vi "HFRR ADV v02.vi"() -> ()   [LabVIEW 2023] (continued)
            n997 = local read "Sample ID"() -> (w2636:string)
            n998 = local read "Temperature after test 2"() -> (w2623:dbl)
            n999 = local read "Test Date"() -> (w2635:string)
            n1000 = local read "String 45"() -> (w2549:string)
            n1001 = local read "String 32"() -> (w2633:string)
            n1002 = local read "String 31"() -> (w2634:string)
            n1003 = local read "String 38"() -> (w2571:string)
            n1004 = local read "Humidity after test 2"() -> (w2619:dbl)
            n1005 = local read "s.NO"() -> (w2551:string)
            n1006 = local read "String 36"() -> (w2574:string)
            n1007 = local read "Temperature before test 2"() -> (w2618:dbl)
            n1008 = local read "String 37"() -> (w2577:string)
            n1009 = local read "AVP 2"() -> (w2616:dbl)
            n1010 = local read "HCF 2"() -> (w2627:dbl)
            n1011 = local read "MWSD 2"() -> (w2615:dbl)
            n1012 = local read "String 35"() -> (w2581:string)
            n1013 = local write "Export"(FALSE ("Export")) -> ()
            n1014 = local read "Humidity before test 2"() -> (w2604:dbl)
            n1015 = Concatenate Strings("7," ("string"), w2571) -> (w2572:string)
            n1016 = Concatenate Strings("6," ("string"), w2574) -> (w2575:string)
            n1017 = local read "S 39"() -> (w2582:string)
            n1018 = Concatenate Strings("5," ("string"), w2577) -> (w2578:string)
            n1019 = local read "String 34"() -> (w2586:string)
            n1020 = Concatenate Strings("4," ("string"), w2581) -> (w2580:string)
            n1021 = Concatenate Strings("3," ("string"), w2582) -> (w2584:string)
            n1022 = local read "S 38"() -> (w2589:string)
            n1023 = Number To Fractional String(number=w2627, width (-)=i16 6, precision (6)=i16 2) -> (F-format string=w2628:string)  [unwired: 1 in]
            n1024 = Number To Fractional String(number=w2615, width (-)=i16 6, precision (6)=i16 2) -> (F-format string=w2613:string)  [unwired: 1 in]
            n1025 = Number To Fractional String(number=w2616, width (-)=i16 6, precision (6)=i16 2) -> (F-format string=w2614:string)  [unwired: 1 in]
            n1026 = Number To Fractional String(number=w2623, width (-)=i16 6, precision (6)=i16 2) -> (F-format string=w2622:string)  [unwired: 1 in]
            n1027 = Number To Fractional String(number=w2619, width (-)=i16 6, precision (6)=i16 2) -> (F-format string=w2617:string)  [unwired: 1 in]
            n1028 = Number To Fractional String(number=w2618, width (-)=i16 6, precision (6)=i16 2) -> (F-format string=w2624:string)  [unwired: 1 in]
            n1029 = Number To Fractional String(number=w2604, width (-)=i16 6, precision (6)=i16 2) -> (F-format string=w2603:string)  [unwired: 1 in]
            n1030 = local read "String 39"() -> (w2568:string)
            n1031 = Concatenate Strings("2," ("string"), w2586) -> (w2585:string)
            n1032 = local read "WS1.4 2"() -> (w2631:dbl)
            n1033 = Concatenate Strings(w2561, "," ("string"), w2549, w2551, w2550, w2633, w2636, w2550, w2634, w2635, w2561) -> (w2559:string)
            n1034 = Concatenate Strings("1," ("string"), w2589) -> (w2588:string)
            n1035 = Concatenate Strings("8," ("string"), w2568) -> (w2569:string)
            n1036 = Number To Fractional String(number=w2631, precision (6)=i16 2) -> (F-format string=w2632:string)  [unwired: 2 in]
            n1037 = Concatenate Strings(w2629, w2588, w2603, w2629, w2585, w2624, w2629, w2584, w2617, w2629, w2580, w2622, w2629, w2578, w2613, w2629, w2575, w2614, w2629, w2572, w2628, w2629, w2569, w2632) -> (w2591:string)
            n1038 = Concatenate Strings("S.No," ("string"), "                                       Parameters" ("string")) -> (w2562:string)
            n1039 = local read "TITTLE"() -> (w2557:string)
            n1040 = local read "String 33"() -> (w2566:string)
            n1041 = local read "Tested by"() -> (w2565:string)
            n1042 = Concatenate Strings("=" ("string"), w2557) -> (w2556:string)
            n1043 = local read "String 29"() -> (w2598:string)
            n1044 = Concatenate Strings("," ("string"), "                                                                             " ("string")) -> (w2554:string)
            n1045 = Concatenate Strings(w2556, w2552, w2559, w2552, w2562, w2591, w2552, w2554, w2566, w2565) -> (→"export":string)
            n1046 = Match Pattern(string=w2598, regular expression=".dwm") -> (before substring=w2594:string)  [unwired: 1 in, 3 out]
            "before substring" <- w2594
            n1047 = case shown="\"xlx\"" "Select File Type" {
              tunnel: w2594 -> [w2639 w2641 w2643]
              tunnel: [w2637 w2642 w2644] -> w2593
              frame "xlx" {
                n1048 = Concatenate Strings(w2639, ".xls" ("string")) -> (w2637:string)
              }
              frame "csv" {
                n1049 = Concatenate Strings(w2641, ".csv" ("string")) -> (w2642:string)
              }
              frame "txt" {
                n1050 = Concatenate Strings(w2643, ".txt" ("string")) -> (w2644:string)
              }
            }
            n1051 = String To Path(string=w2593) -> (path=w2600:path)
            n1052 = local read "export"() -> (w2595:string)
            n1053 = call <vilib>:"Write Characters To File.vi"("append to file? (new file:F)"=FALSE, "character string"=w2595, "file path (dialog if empty)"=w2600) -> ()  [unwired: 2 in, 1 out]
          }
        }
        n1054 = case shown="True" "OK Button 16" {
          frame False {
          }
          frame True {
            n1055 = stacked-sequence {
              frame #0 {
                n1056 = local read "Numeric 16"() -> (w2759:i32)
                n1057 = local write "Numeric 10"(w2759) -> ()
              }
              frame #1 {
                n1058 = local read "String 29"() -> (w2763:string)
                n1059 = String To Path(string=w2763) -> (path=w2762:path)
                n1060 = local read "S.NO"() -> (→"s.NO":string)
                n1061 = Open/Create/Replace File "Open File"(file path (use dialog)=w2762) -> (refnum out=w2764:refnum<file>)  [unwired: 5 in, 2 out]
                n1062 = for {
                  N: 16 -> [_]
                  tunnel: w2764 -> [w2771]
                  i -> [w2767]
                  (unwired) TRUE ("line mode (F)")
                  n1063 = Read from Text File "Read File"(file (use dialog)=w2771) -> (text=w2765:string)  [unwired: 3 in, 3 out]
                  n1064 = Match Pattern(string=w2765, regular expression="(") -> (after substring=w2770:string)  [unwired: 1 in, 3 out]
                  n1065 = Match Pattern(string=w2770, regular expression=")") -> (before substring=w2766:string)  [unwired: 1 in, 3 out]
                  n1066 = case shown="1" w2767 {
                    tunnel: w2766 -> [w2772 w2773 _ _ w2774 w2775 w2776 w2778 w2780 w2782 w2784 w2786 w2788 w2790 _]
                    tunnel: w2765 -> [_ _ _ _ _ _ _ _ _ _ _ _ _ _ _]
                    frame 0 {
                      "TITTLE" <- w2772
                    }
                    frame 1 {
                      "Sample ID" <- w2773
                    }
                    frame 2 {
                    }
                    frame 3 {
                    }
                    frame 4 {
                      "Test Date" <- w2774
                    }
                    frame 5 {
                      "Tested by" <- w2775
                    }
                    frame 6 {
                      n1067 = Fract/Exp String To Number(string=w2776) -> (number=→"Humidity before test 2":dbl)  [unwired: 3 in, 1 out]
                    }
                    frame 7 {
                      n1068 = Fract/Exp String To Number(string=w2778) -> (number=→"Temperature before test 2":dbl)  [unwired: 3 in, 1 out]
                    }
                    frame 8 {
                      n1069 = Fract/Exp String To Number(string=w2780) -> (number=→"Humidity after test 2":dbl)  [unwired: 3 in, 1 out]
                    }
                    frame 9 {
                      n1070 = Fract/Exp String To Number(string=w2782) -> (number=→"Temperature after test 2":dbl)  [unwired: 3 in, 1 out]
                    }
                    frame 10 {
                      n1071 = Fract/Exp String To Number(string=w2784) -> (number=→"MWSD 2":dbl)  [unwired: 3 in, 1 out]
                    }
                    frame 11 {
                      n1072 = Fract/Exp String To Number(string=w2786) -> (number=→"AVP 2":dbl)  [unwired: 3 in, 1 out]
                    }
                    frame 12 {
                      n1073 = Fract/Exp String To Number(string=w2788) -> (number=→"HCF 2":dbl)  [unwired: 3 in, 1 out]
                    }
                    frame 13 {
                      n1074 = Fract/Exp String To Number(string=w2790) -> (number=→"WS1.4 2":dbl)  [unwired: 3 in, 1 out]
                    }
                    frame 14, Default {
                    }
                  }
                }
              }
              frame #2 {
              }
            }
            n1075 = local write "OK Button 16"(FALSE ("OK Button 13")) -> ()
          }
        }
        n1076 = call <vilib>:"Query Available Printers.vi"() -> ("system configured printers"=w2434:string[])  [unwired: 9 in, 2 out]
        "System Configured Printers 2" <- w2434
        n1077 = Index Array(array=w2434, index="Select Printer 3") -> (element=w2436:string)
        "Selected Printer" <- w2436
        n1078 = local read "OK Button 16"() -> (w2430:bool)
        n1079 = case shown="True" "Print" {
          tunnel: w2436 -> [_ w2728]
          frame False {
          }
          frame True {
            (unwired) i16 6 ("width (-)")
            (unwired) "TESTED BY : "
            (unwired) "TESTED DATE :"
            (unwired) "SAMPLE ID : "
            (unwired) "SAMPLE DESIGN : "
            w2686 = "\r"
            w2703 = "\r"
            # "add image"
            n1080 = local read "String 45"() -> (w2646:string)
            n1081 = local read "Sample ID"() -> (w2676:string)
            n1082 = local read "Tested by"() -> (w2679:string)
            n1083 = local read "Test Date"() -> (w2677:string)
            n1084 = local read "String 32"() -> (w2681:string)
            n1085 = local read "String 31"() -> (w2680:string)
            n1086 = local read "String 33"() -> (w2682:string)
            n1087 = local read "s.NO"() -> (w2647:string)
            n1088 = call <vilib>:"New Report.vi"("report type"=enum16{"Standard Report", "HTML"}."Standard Report") -> ("report out"=w2726:refnum<class "NI_report.lvclass">, "error out"=w2725:errorcluster)  [unwired: 13 in]
            n1089 = local read "TITTLE"() -> (w2678:string)
            n1090 = call-dynamic "Set Report Header Text.vi"("report in"=w2726, "center header text"=w2678, "error in (no error)"=w2725) -> ("report out"=w2697:refnum<class "NI_report.lvclass">, "error out"=w2698:errorcluster)  [unwired: 11 in]
            n1091 = Concatenate Strings(w2703, w2646, w2647, w2703, w2681, w2676, w2703, w2680, w2677, w2703, w2682, w2679, w2703) -> (w2696:string)
            "test by" <- w2696
            n1092 = local read "Temperature after test 2"() -> (w2692:dbl)
            n1093 = local read "String 38"() -> (w2652:string)
            n1094 = local read "Humidity after test 2"() -> (w2701:dbl)
            n1095 = local read "String 36"() -> (w2656:string)
            n1096 = local read "Temperature before test 2"() -> (w2702:dbl)
            n1097 = local read "String 37"() -> (w2659:string)
            n1098 = local read "AVP 2"() -> (w2705:dbl)
            n1099 = local read "HCF 2"() -> (w2688:dbl)
            n1100 = local read "MWSD 2"() -> (w2706:dbl)
            n1101 = local read "String 35"() -> (w2661:string)
            n1102 = call-poly <vilib>:"Append Report Text.vi"("report in"=w2697, "text"=w2696, "error in (no error)"=w2698) -> ("report out"=w2700:refnum<class "NI_report.lvclass">, "error out"=w2699:errorcluster)  [unwired: 9 in, 2 out]
            n1103 = local read "Humidity before test 2"() -> (w2717:dbl)
            n1104 = Concatenate Strings("7)" ("string"), w2652) -> (w2653:string)
            n1105 = local read "S 39"() -> (w2664:string)
            n1106 = local read "String 34"() -> (w2666:string)
            n1107 = Concatenate Strings("6)" ("string"), w2656) -> (w2655:string)
            n1108 = Concatenate Strings("5)" ("string"), w2659) -> (w2658:string)
            n1109 = Concatenate Strings("4)" ("string"), w2661) -> (w2662:string)
            n1110 = Concatenate Strings("3)" ("string"), w2664) -> (w2665:string)
            n1111 = local read "S 38"() -> (w2671:string)
            n1112 = Concatenate Strings("2)" ("string"), w2666) -> (w2667:string)
            n1113 = Number To Fractional String(number=w2688, width (-)=i16 6, precision (6)=i16 2) -> (F-format string=w2687:string)  [unwired: 1 in]
            n1114 = Number To Fractional String(number=w2706, width (-)=i16 6, precision (6)=i16 2) -> (F-format string=w2708:string)  [unwired: 1 in]
            n1115 = Number To Fractional String(number=w2705, width (-)=i16 6, precision (6)=i16 2) -> (F-format string=w2707:string)  [unwired: 1 in]
            n1116 = Number To Fractional String(number=w2692, width (-)=i16 6, precision (6)=i16 2) -> (F-format string=w2693:string)  [unwired: 1 in]
            n1117 = Number To Fractional String(number=w2701, width (-)=i16 6, precision (6)=i16 2) -> (F-format string=w2704:string)  [unwired: 1 in]
            n1118 = Number To Fractional String(number=w2702, width (-)=i16 6, precision (6)=i16 2) -> (F-format string=w2691:string)  [unwired: 1 in]
            n1119 = Number To Fractional String(number=w2717, width (-)=i16 6, precision (6)=i16 2) -> (F-format string=w2722:string)  [unwired: 1 in]
            n1120 = call-poly <vilib>:"Append Report Text.vi"("report in"=w2700, "error in (no error)"=w2699) -> ("report out"=w2721:refnum<class "NI_report.lvclass">, "error out"=w2719:errorcluster)  [unwired: 10 in, 2 out]
            n1121 = local read "String 39"() -> (w2649:string)
            n1122 = local read "WS1.4 2"() -> (w2684:dbl)
            n1123 = Concatenate Strings("1)" ("string"), w2671) -> (w2670:string)
            n1124 = Concatenate Strings("8)" ("string"), w2649) -> (w2650:string)
            n1125 = Number To Fractional String(number=w2684, precision (6)=i16 2) -> (F-format string=w2683:string)  [unwired: 2 in]
            n1126 = Concatenate Strings(w2686, w2670, w2722, w2686, w2667, w2691, w2686, w2665, w2704, w2686, w2662, w2693, w2686, w2658, w2708, w2686, w2655, w2707, w2686, w2653, w2687, w2686, w2650, w2683) -> (w2674:string)
            "export 2" <- w2674
            n1127 = call-poly <vilib>:"Append Report Text.vi"("report in"=w2721, "text"=w2674, "error in (no error)"=w2719) -> ("report out"=w2720:refnum<class "NI_report.lvclass">, "error out"=w2718:errorcluster)  [unwired: 9 in, 2 out]
            n1128 = call-dynamic "Print Report.vi"("report in"=w2720, "printer name (default)"=w2728, "error in (no error)"=w2718) -> ("report out"=w2730:refnum<class "NI_report.lvclass">, "error out"=w2731:errorcluster)  [unwired: 11 in]
            n1129 = local read "test by"() -> (w2673:string)
            n1130 = local read "TITTLE"() -> (w2675:string)
            n1131 = local write "Print"(FALSE ("Print FF")) -> ()
            n1132 = call-dynamic "Dispose Report.vi"("report in"=w2730, "error in (no error)"=w2731) -> ()  [unwired: 13 in, 1 out]
            n1133 = Concatenate Strings(w2675, w2674, w2673) -> (→"output":string)
          }
        }
        n1134 = case shown="True" w2430 {
          frame False {
          }
          frame True {
            n1135 = flat-sequence {
              frame #0 {
              }
              frame #1 {
                n1136 = Wait (ms)(milliseconds to wait=u32 100) -> ()  [unwired: 1 out]
              }
              frame #2 {
                n1137 = local write "OK Button 16"(FALSE ("Print 3")) -> ()
              }
            }
          }
        }
        n1138 = case shown="True" "OK Button 17" {
          frame False {
          }
          frame True {
            (unwired) 0  # existing file
            w2745 = "Choose a datalog file to open"  # prompt
            n1139 = local read "String"() -> (w2740:string)
            n1140 = local write "OK Button 17"(FALSE ("OK Button 17")) -> ()
            n1141 = String To Path(string=w2740) -> (path=w2741:path)
            n1142 = File Dialog(6:"*.duf" ("pattern"), 7:w2745, 11:w2741) -> (0:w2732:errorcluster, 3:w2751:path)  [unwired: 4 in, 2 out]
            n1143 = Unbundle(w2732) -> ()  [unwired: 3 out]
            n1144 = Open/Create/Replace File "Open File"(file path (use dialog)=w2751) -> (refnum out=w2743:refnum<file>)  [unwired: 5 in, 2 out]
            n1145 = Path To String(path=w2751) -> (string=w2734:string)
            n1146 = while {
              tunnel: w2743 -> [w2755]
              i -> [w2752]
              stop <- w2753 continue-if-true
              (unwired) TRUE ("line mode (F)")
              n1147 = local write "Numeric 16"(w2752) -> ()
              n1148 = Read from Text File "Read File"(file (use dialog)=w2755) -> (text=w2754:string)  [unwired: 3 in, 3 out]
              n1149 = String Length(string=w2754) -> (length=w2757:i32)
              n1150 = Greater?(x=w2757, y=1) -> (0:w2753:bool)
            }
            n1151 = local write "String 29"(w2734) -> ()
            n1152 = Match Pattern(string=w2734, regular expression=".dwm" ("substring (\"\")")) -> (before substring=w2735:string)  [unwired: 1 in, 3 out]
            "String Indicator 3" <- w2735
            n1153 = Search and Replace String(input string=w2734, search string=".duf", replace string=".dgf" ("replace string (\"\")")) -> (result string=→"String Indicator 4":string)  [unwired: 5 in, 3 out]
            n1154 = String To Path(string=w2735) -> (path=w2742:path)
            "path" <- w2742
            n1155 = Strip Path(path=w2751) -> (name=w2749:string)  [unwired: 1 out]
            n1156 = call <vilib>:"Read Characters From File.vi"("file path (dialog if empty)"=w2742, "start of read offset (chars.:0)"=60 ("start of read offset (chars.: 0)")) -> ("character string"=→"String Indicator 2":string)  [unwired: 4 in, 3 out]
            n1157 = Match Pattern(string=w2749, regular expression=".dwm") -> (before substring=w2733:string)  [unwired: 1 in, 3 out]
            "String Indicator" <- w2733
            n1158 = local write "TITTLE 2"(w2733) -> ()
          }
        }
        n1159 = case shown="True" "Print 2" {
          frame False {
          }
          frame True {
            n1160 = flat-sequence {
              frame #0 {
                n1161 = local read "Ref A Test Date :"() -> (→"TITTLE 4":string)
                n1162 = local read "Sample ID"() -> (→"Sample ID  2":string)
                n1163 = local read "s.NO"() -> (→"s.NO 2":string)
                n1164 = local read "Test Date"() -> (→"Test Date 2":string)
                n1165 = local read "Tested by"() -> (→"Tested by 2":string)
                n1166 = local read "Temperature before test 3"() -> (w2454:dbl)
                n1167 = local read "Temperature before test 3"() -> (→"Temperature after test 5":dbl)
                n1168 = local read "Temperature after test 3"() -> (→"Temperature after test 4":dbl)
                n1169 = local read "Sample ID  3"() -> (→"Sample ID  6":string)
                n1170 = local read "Sample ID  4"() -> (→"Sample ID  7":string)
                n1171 = local read "Humidity before test 3"() -> (→"Humidity before test 4":dbl)
                n1172 = local read "Humidity after test 3"() -> (→"Humidity after test 4":dbl)
                n1173 = local write "Temperature before test 3"(w2454) -> ()
                n1174 = String To Path(string="C:\\LAB-IQ-NXT\\im\\Temp_resized.jpg") -> (path=w2446:path)
                "path 2" <- w2446
                n1175 = local read "image data"() -> (w2445:T8)
                n1176 = Wait (ms)(milliseconds to wait=u32 20) -> ()  [unwired: 1 out]
                n1177 = call <vilib>:"Write JPEG File.vi"("image data"=w2445, "path to JPEG file"=w2446) -> ()  [unwired: 8 in, 2 out]
                "Ref A Test Date :" <- "Ref A Test Date :"
                "Ref B Test Date :" <- "Ref B Test Date :"
                "Ref B Scar Value :" <- "Ref B Scar Value :"
                "Ref A Scar Value :" <- "Ref A Scar Value :"
              }
              frame #1 {
                (unwired) HTML_Report_Image_Alignment."MIDDLE" ("alignment (default)")
                w2482 = u16 0 items=["portrait", "landscape"] ("orientation (portrait)")
                (unwired) HTML_Report_Image_Alignment."ABSMIDDLE" ("alignment (default)")
                (unwired) "TESTED BY : "
                (unwired) "TESTED DATE :"
                (unwired) "SAMPLE ID : "
                (unwired) "SAMPLE DESIGN : "
                w2515 = "\r"
                # "add image"
                n1178 = call <vilib>:"New Report.vi"("report type"=enum16{"Standard Report", "HTML"}."HTML") -> ("report out"=w2486:refnum<class "NI_report.lvclass">, "error out"=w2484:errorcluster)  [unwired: 13 in]
                n1179 = Wait (ms)(milliseconds to wait=u32 20) -> ()  [unwired: 1 out]
                n1180 = call-dynamic "Set Report Orientation.vi"("report in"=w2486, "orientation (portrait)"=w2482, "error in (no error)"=w2484) -> ("report out"=w2485:refnum<class "NI_report.lvclass">, "error out"=w2483:errorcluster)  [unwired: 11 in]
                n1181 = for {
                  N: 5 -> [_]
                  tunnel: w2485 -> [w2536]
                  tunnel: [w2535] -> w2464
                  tunnel: w2483 -> [w2534]
                  tunnel: [w2533] -> w2463
                  n1182 = call-dynamic "Set Report Tab Width.vi"("report in"=w2536, "error in (no error)"=w2534) -> ("report out"=w2535:refnum<class "NI_report.lvclass">, "error out"=w2533:errorcluster)  [unwired: 12 in]
                }
                n1183 = local read "Sample ID  2"() -> (w2508:string)
                n1184 = local read "s.NO 2"() -> (w2507:string)
                n1185 = local read "Test Date 2"() -> (w2509:string)
                n1186 = local read "Tested by 2"() -> (w2510:string)
                n1187 = local read "String 46"() -> (w2506:string)
                n1188 = local read "String 48"() -> (w2512:string)
                n1189 = local read "String 47"() -> (w2511:string)
                n1190 = local read "String 49"() -> (w2513:string)
                n1191 = local read "TITTLE"() -> (w2481:string)
                n1192 = call-dynamic "Set Report Header Text.vi"("report in"=w2464, "center header text"=w2481, "error in (no error)"=w2463) -> ("report out"=w2502:refnum<class "NI_report.lvclass">, "error out"=w2501:errorcluster)  [unwired: 11 in]
                n1193 = for {
                  N: 1 -> [_]
                  tunnel: [w2540] -> w2488
                  tunnel: [w2539] -> w2487
                  tunnel: w2502 -> [w2538]
                  tunnel: w2501 -> [w2537]
                  n1194 = call-dynamic "New Report Line.vi"("report in"=w2538, "error in (no error)"=w2537) -> ("report out"=w2540:refnum<class "NI_report.lvclass">, "error out"=w2539:errorcluster)  [unwired: 12 in]
                }
                n1195 = for {
                  N: 2 -> [_]
                  tunnel: [w2532] -> w2494
                  tunnel: [w2531] -> w2493
                  tunnel: w2488 -> [w2530]
                  tunnel: w2487 -> [w2529]
                  n1196 = call-dynamic "New Report Line.vi"("report in"=w2530, "error in (no error)"=w2529) -> ("report out"=w2532:refnum<class "NI_report.lvclass">, "error out"=w2531:errorcluster)  [unwired: 12 in]
                }
                n1197 = Concatenate Strings(w2515, w2506, w2507, w2515, w2512, w2508, w2515, w2511, w2509, w2515, w2513, w2510, w2515) -> (→"test by 2":string)
                n1198 = for {
                  N: 25 -> [_]
                  tunnel: w2494 -> [w2528]
                  tunnel: w2493 -> [w2526]
                  tunnel: [w2527] -> w2497
                  tunnel: [w2525] -> w2496
                  n1199 = call-dynamic "Set Report Tab Width.vi"("report in"=w2528, "error in (no error)"=w2526) -> ("report out"=w2527:refnum<class "NI_report.lvclass">, "error out"=w2525:errorcluster)  [unwired: 12 in]
                }
                n1200 = control-ref of="Tab Control 9"() -> (w2492:refnum<vi>)
                n1201 = local read "Wear Scar X"() -> (w2480:dbl)
                "Length ( microns ) 2" <- w2480
                n1202 = local read "Wear Scar Y"() -> (w2479:dbl)
                "Wear Scar Y ( microns ) :" <- w2479
                n1203 = call-dynamic "Append Control Image to Report.vi"("report in"=w2497, "alignment (default)"=HTML_Report_Image_Alignment."ABSMIDDLE", "ctrl reference"=w2492, "error in (no error)"=w2496) -> ("report out"=w2491:refnum<class "NI_report.lvclass">, "error out"=w2490:errorcluster)  [unwired: 8 in, 2 out]
                n1204 = for {
                  N: 3 -> [_]
                  tunnel: [w2524] -> w2475
                  tunnel: [w2523] -> w2474
                  tunnel: w2491 -> [w2522]
                  tunnel: w2490 -> [w2521]
                  n1205 = call-dynamic "New Report Line.vi"("report in"=w2522, "error in (no error)"=w2521) -> ("report out"=w2524:refnum<class "NI_report.lvclass">, "error out"=w2523:errorcluster)  [unwired: 12 in]
                }
                n1206 = Add(x=w2480, y=w2479) -> (x+y=w2478:dbl)
                n1207 = Divide(x=w2478, y=2.0) -> (x/y=→"Mean Wear ( microns) :":dbl)
                n1208 = for {
                  N: 100 -> [_]
                  tunnel: w2475 -> [w2520]
                  tunnel: w2474 -> [w2518]
                  tunnel: [w2519] -> w2471
                  tunnel: [w2517] -> w2469
                  n1209 = call-dynamic "Set Report Tab Width.vi"("report in"=w2520, "error in (no error)"=w2518) -> ("report out"=w2519:refnum<class "NI_report.lvclass">, "error out"=w2517:errorcluster)  [unwired: 12 in]
                }
                n1210 = local read "String 10"() -> (w2466:string)
                n1211 = Concatenate Strings("C:\\LAB-IQ-NXT\\Data\\" ("string"), w2466, ".jpg" ("string")) -> ()  [unwired: 1 out]
                n1212 = String To Path(string="C:\\LAB-IQ-NXT\\im\\Temp_resized.jpg") -> (path=w2461:path)
                n1213 = call-poly <vilib>:"Append Image to Report.vi"("report in"=w2471, "path or URL of image"=w2461, "error in (no error)"=w2469) -> ("report out"=w2470:refnum<class "NI_report.lvclass">, "error out"=w2468:errorcluster)  [unwired: 9 in, 2 out]
                n1214 = call-poly <vilib>:"Open HTML Report in Browser.vi"("report in"=w2470, "error in (no error)"=w2468) -> ("report out"=w2505:refnum<class "NI_report.lvclass">, "error out"=w2504:errorcluster)  [unwired: 11 in, 1 out]
                n1215 = call-dynamic "Dispose Report.vi"("report in"=w2505, "error in (no error)"=w2504) -> ()  [unwired: 13 in, 1 out]
              }
              frame #2 {
              }
              frame #3 {
                n1216 = case shown="True" "Case Constant\n(See Context Help) 16" {
                  frame False {
                  }
                  frame True {
                    n1217 = local read "String 10"() -> (w2546:string)
                    n1218 = Concatenate Strings("C:\\LAB-IQ-NXT\\Data\\" ("string"), w2546, ".jpg" ("string")) -> (w2544:string)
                    n1219 = String To Path(string=w2544) -> (path=w2543:path)
                    n1220 = Delete(path (use dialog)=w2543) -> ()  [unwired: 4 in, 3 out]
                  }
                }
                n1221 = local write "Print 2"(FALSE ("Print")) -> ()
              }
            }
          }
        }
      }
    }
    n1222 = local read "OK Button 16"() -> (w788:bool)
    n1223 = Or(x=w788, y="OPEN") -> (x .or. y?=w789:bool)
    n1224 = case shown="True" w789 {
      tunnel: w788 -> [_ w841]
      frame False {
      }
      frame True {
        n1225 = stacked-sequence {
          tunnel: w841 -> [_ w908 _ _]
          frame #0 {
            w857 = "  " ("String 6")
            n1226 = local write "OPEN"(FALSE ("open")) -> ()
            n1227 = property on="OPEN" class="Bool (strict)"("Visible"=FALSE) -> ()  [unwired: 2 in, 2 out]
            n1228 = local write "String 12"(w857) -> ()
            n1229 = local write "String 6"(w857) -> ()
            n1230 = local write "String 7"(w857) -> ()
            n1231 = local write "String 8"(w857) -> ()
            n1232 = local read "OK Button 16"() -> (w842:bool)
            n1233 = case shown="True" w842 {
              tunnel: [w858 w859] -> w846
              frame False {
                n1234 = local read "string1"() -> (w858:string)
              }
              frame True {
                n1235 = local read "String Indicator 4"() -> (w859:string)
              }
            }
            n1236 = local read "string1 2"() -> (w845:string)
            n1237 = local read "string1 4"() -> (w843:string)
            n1238 = local read "string1 3"() -> (w844:string)
            n1239 = String To Path(string=w846) -> (path=w854:path)
            n1240 = String To Path(string=w845) -> (path=w853:path)
            n1241 = String To Path(string=w844) -> (path=w852:path)
            n1242 = String To Path(string=w843) -> (path=w851:path)
            n1243 = Open/Create/Replace File "Open File"(file path (use dialog)=w854) -> (refnum out=w850:refnum<file>)  [unwired: 5 in, 2 out]
            n1244 = Open/Create/Replace File "Open File"(file path (use dialog)=w853) -> (refnum out=w849:refnum<file>)  [unwired: 5 in, 2 out]
            n1245 = Open/Create/Replace File "Open File"(file path (use dialog)=w852) -> (refnum out=w848:refnum<file>)  [unwired: 5 in, 2 out]
            n1246 = Open/Create/Replace File "Open File"(file path (use dialog)=w851) -> (refnum out=w847:refnum<file>)  [unwired: 5 in, 2 out]
            n1247 = while {
              tunnel: w850 -> [w865]
              i -> [w861]
              stop <- w860 continue-if-true
              (unwired) TRUE ("line mode (F)")
              n1248 = Read from Text File "Read File"(file (use dialog)=w865) -> (text=w862:string)  [unwired: 3 in, 3 out]
              n1249 = local write "Numeric 8"(w861) -> ()
              n1250 = String Length(string=w862) -> (length=w864:i32)
              n1251 = Greater?(x=w864, y=1) -> (0:w860:bool)
            }
            n1252 = while {
              tunnel: w849 -> [w871]
              i -> [w867]
              stop <- w866 continue-if-true
              (unwired) TRUE ("line mode (F)")
              n1253 = Read from Text File "Read File"(file (use dialog)=w871) -> (text=w868:string)  [unwired: 3 in, 3 out]
              n1254 = local write "Numeric 11"(w867) -> ()
              n1255 = String Length(string=w868) -> (length=w870:i32)
              n1256 = Greater?(x=w870, y=1) -> (0:w866:bool)
            }
            n1257 = while {
              tunnel: w848 -> [w877]
              i -> [w873]
              stop <- w872 continue-if-true
              (unwired) TRUE ("line mode (F)")
              n1258 = Read from Text File "Read File"(file (use dialog)=w877) -> (text=w874:string)  [unwired: 3 in, 3 out]
              n1259 = local write "Numeric 12"(w873) -> ()
              n1260 = String Length(string=w874) -> (length=w876:i32)
              n1261 = Greater?(x=w876, y=1) -> (0:w872:bool)
            }
            n1262 = while {
              tunnel: w847 -> [w883]
              i -> [w879]
              stop <- w878 continue-if-true
              (unwired) TRUE ("line mode (F)")
              n1263 = Read from Text File "Read File"(file (use dialog)=w883) -> (text=w880:string)  [unwired: 3 in, 3 out]
              n1264 = local write "Numeric 13"(w879) -> ()
              n1265 = String Length(string=w880) -> (length=w882:i32)
              n1266 = Greater?(x=w882, y=1) -> (0:w878:bool)
            }
          }
          frame #1 {
            w1035 = FALSE ("ACTUAL   MERGE")
            # "Sample Temp"
            # "ECR"
            # "COF"
            # "Time\nCOF\nFF\nTemp"
            n1267 = case shown="True" w908 {
              tunnel: [w1055 w1056] -> w909
              frame False {
                n1268 = local read "string1"() -> (w1055:string)
              }
              frame True {
                n1269 = local read "String Indicator 4"() -> (w1056:string)
              }
            }
            n1270 = local read "string1 2"() -> (w954:string)
            n1271 = local read "string1 4"() -> (w952:string)
            n1272 = local read "string1 3"() -> (w953:string)
            n1273 = String To Path(string=w952) -> (path=w1046:path)
            n1274 = String To Path(string=w954) -> (path=w1052:path)
            n1275 = String To Path(string=w909) -> (path=w1040:path)
            n1276 = Open/Create/Replace File "Open File"(file path (use dialog)=w1046) -> (refnum out=w1045:refnum<file>, error out=w1044:errorcluster)  [unwired: 5 in, 1 out]
            n1277 = Open/Create/Replace File "Open File"(file path (use dialog)=w1040) -> (refnum out=w1054:refnum<file>, error out=w1053:errorcluster)  [unwired: 5 in, 1 out]
            n1278 = Open/Create/Replace File "Open File"(file path (use dialog)=w1052) -> (refnum out=w1050:refnum<file>, error out=w1049:errorcluster)  [unwired: 5 in, 1 out]
            n1279 = String To Path(string=w953) -> (path=w1051:path)
            n1280 = local read "Numeric 8"() -> (w1039:i32)
            n1281 = Open/Create/Replace File "Open File"(file path (use dialog)=w1051) -> (refnum out=w1047:refnum<file>, error out=w1048:errorcluster)  [unwired: 5 in, 1 out]
            n1282 = local read "Numeric 13"() -> (w1038:i32)
            n1283 = local read "Numeric 11"() -> (w1036:i32)
            n1284 = local read "Numeric 12"() -> (w1037:i32)
            n1285 = for {
              N: w1036 -> [_]
              tunnel: w1050 -> [w1165]
              tunnel: w1049 -> [w1164]
              tunnel: [w1154] -> w1016 mode=indexing
              tunnel: [w1152] -> w1014 mode=indexing
              tunnel: [w1153] -> w1009 mode=indexing
              tunnel: w1035 -> [_]
              tunnel: [w1146] -> w1011 mode=indexing
              tunnel: [w1142] -> w987 mode=indexing
              tunnel: [w1138] -> w962 mode=indexing
              tunnel: [w1134] -> w943 mode=indexing
              tunnel: [w1129] -> w901 mode=indexing
              (unwired) TRUE ("line mode (F)")
              n1286 = Read from Text File "Read File"(file (use dialog)=w1165, error in=w1164) -> (text=w1130:string)  [unwired: 2 in, 3 out]
              n1287 = String Subset(string=w1130, offset (0)=0, length (rest)=14 ("length (rest)")) -> (substring=w1158:string)
              n1288 = Fract/Exp String To Number(string=w1158) -> (number=w1154:dbl)  [unwired: 3 in, 1 out]
              n1289 = local write "String 7"(w1130) -> ()
              n1290 = String Subset(string=w1130, offset (0)=15, length (rest)=9 ("length (rest)")) -> (substring=w1161:string)
              n1291 = Fract/Exp String To Number(string=w1161) -> (number=w1152:dbl)  [unwired: 3 in, 1 out]
              n1292 = String Subset(string=w1130, offset (0)=65, length (rest)=9 ("length (rest)")) -> (substring=w1147:string)
              n1293 = Fract/Exp String To Number(string=w1147) -> (number=w1150:dbl)  [unwired: 3 in, 1 out]
              n1294 = Add(x=w1150, y=0.0) -> (x+y=w1146:dbl)
              n1295 = String Subset(string=w1130, offset (0)=35, length (rest)=9 ("length (rest)")) -> (substring=w1155:string)
              n1296 = Fract/Exp String To Number(string=w1155) -> (number=w1153:dbl)  [unwired: 3 in, 1 out]
              n1297 = String Subset(string=w1130, offset (0)=45, length (rest)=9 ("length (rest)")) -> (substring=w1143:string)
              n1298 = Fract/Exp String To Number(string=w1143) -> (number=w1142:dbl)  [unwired: 3 in, 1 out]
              n1299 = String Subset(string=w1130, offset (0)=55, length (rest)=9 ("length (rest)")) -> (substring=w1141:string)
              n1300 = Fract/Exp String To Number(string=w1141) -> (number=w1138:dbl)  [unwired: 3 in, 1 out]
              n1301 = String Subset(string=w1130, offset (0)=25, length (rest)=9 ("length (rest)")) -> (substring=w1135:string)
              n1302 = Fract/Exp String To Number(string=w1135) -> (number=w1134:dbl)  [unwired: 3 in, 1 out]
              n1303 = String Subset(string=w1130, offset (0)=85, length (rest)=9 ("length (rest)")) -> (substring=w1133:string)
              n1304 = Fract/Exp String To Number(string=w1133) -> (number=w1129:dbl)  [unwired: 3 in, 1 out]
            }
            n1305 = for {
              N: w1037 -> [_]
              tunnel: w1048 -> [w1128]
              tunnel: w1047 -> [w1127]
              tunnel: [w1117] -> w1006 mode=indexing
              tunnel: [w1115] -> w1004 mode=indexing
              tunnel: [w1116] -> w1000 mode=indexing
              tunnel: w1035 -> [_]
              tunnel: [w1109] -> w1002 mode=indexing
              tunnel: [w1105] -> w984 mode=indexing
              tunnel: [w1101] -> w960 mode=indexing
              tunnel: [w1098] -> w941 mode=indexing
              tunnel: [w1094] -> w900 mode=indexing
              (unwired) 9 ("length (rest)")
              (unwired) 9 ("length (rest)")
              (unwired) TRUE ("line mode (F)")
              n1306 = Read from Text File "Read File"(file (use dialog)=w1127, error in=w1128) -> (text=w1095:string)  [unwired: 2 in, 3 out]
              n1307 = String Subset(string=w1095, offset (0)=0, length (rest)=14 ("length (rest)")) -> (substring=w1121:string)
              n1308 = Fract/Exp String To Number(string=w1121) -> (number=w1117:dbl)  [unwired: 3 in, 1 out]
              n1309 = local write "String 8"(w1095) -> ()
              n1310 = String Subset(string=w1095, offset (0)=15, length (rest)=9 ("length (rest)")) -> (substring=w1124:string)
              n1311 = Fract/Exp String To Number(string=w1124) -> (number=w1115:dbl)  [unwired: 3 in, 1 out]
              n1312 = String Subset(string=w1095, offset (0)=65, length (rest)=9 ("length (rest)")) -> (substring=w1114:string)
              n1313 = Fract/Exp String To Number(string=w1114) -> (number=w1111:dbl)  [unwired: 3 in, 1 out]
              n1314 = Add(x=w1111, y=0.0) -> (x+y=w1109:dbl)
              n1315 = String Subset(string=w1095, offset (0)=35, length (rest)=9 ("length (rest)")) -> (substring=w1118:string)
              n1316 = Fract/Exp String To Number(string=w1118) -> (number=w1116:dbl)  [unwired: 3 in, 1 out]
              n1317 = String Subset(string=w1095, offset (0)=45, length (rest)=9 ("length (rest)")) -> (substring=w1108:string)
              n1318 = Fract/Exp String To Number(string=w1108) -> (number=w1105:dbl)  [unwired: 3 in, 1 out]
              n1319 = String Subset(string=w1095, offset (0)=55, length (rest)=9 ("length (rest)")) -> (substring=w1103:string)
              n1320 = Fract/Exp String To Number(string=w1103) -> (number=w1101:dbl)  [unwired: 3 in, 1 out]
              n1321 = String Subset(string=w1095, offset (0)=25) -> (substring=w1099:string)  [unwired: 1 in]
              n1322 = Fract/Exp String To Number(string=w1099) -> (number=w1098:dbl)  [unwired: 3 in, 1 out]
              n1323 = String Subset(string=w1095, offset (0)=85) -> (substring=w1097:string)  [unwired: 1 in]
              n1324 = Fract/Exp String To Number(string=w1097) -> (number=w1094:dbl)  [unwired: 3 in, 1 out]
            }
            n1325 = for {
              N: w1038 -> [_]
              tunnel: w1045 -> [w1093]
              tunnel: w1044 -> [w1092]
              tunnel: [w1082] -> w998 mode=indexing
              tunnel: [w1081] -> w991 mode=indexing
              tunnel: w1035 -> [_]
              tunnel: [w1070] -> w996 mode=indexing
              tunnel: [w1075] -> w993 mode=indexing
              tunnel: [w1071] -> w983 mode=indexing
              tunnel: [w1066] -> w958 mode=indexing
              tunnel: [w1062] -> w939 mode=indexing
              tunnel: [w1057] -> w899 mode=indexing
              (unwired) 1.0 ("x")
              (unwired) TRUE ("line mode (F)")
              n1326 = Read from Text File "Read File"(file (use dialog)=w1093, error in=w1092) -> (text=w1058:string)  [unwired: 2 in, 3 out]
              n1327 = String Subset(string=w1058, offset (0)=0, length (rest)=14 ("length (rest)")) -> (substring=w1086:string)
              n1328 = Fract/Exp String To Number(string=w1086) -> (number=w1082:dbl)  [unwired: 3 in, 1 out]
              n1329 = String Subset(string=w1058, offset (0)=15, length (rest)=9 ("length (rest)")) -> (substring=w1089:string)
              n1330 = local write "String 12"(w1058) -> ()
              n1331 = Fract/Exp String To Number(string=w1089) -> (number=w1070:dbl)  [unwired: 3 in, 1 out]
              n1332 = String Subset(string=w1058, offset (0)=65, length (rest)=9 ("length (rest)")) -> (substring=w1076:string)
              n1333 = Fract/Exp String To Number(string=w1076) -> (number=w1079:dbl)  [unwired: 3 in, 1 out]
              n1334 = Add(x=w1079, y=0.0) -> (x+y=w1075:dbl)
              n1335 = String Subset(string=w1058, offset (0)=35, length (rest)=9 ("length (rest)")) -> (substring=w1083:string)
              n1336 = Fract/Exp String To Number(string=w1083) -> (number=w1081:dbl)  [unwired: 3 in, 1 out]
              n1337 = String Subset(string=w1058, offset (0)=45, length (rest)=9 ("length (rest)")) -> (substring=w1073:string)
              n1338 = Fract/Exp String To Number(string=w1073) -> (number=w1071:dbl)  [unwired: 3 in, 1 out]
              n1339 = String Subset(string=w1058, offset (0)=55, length (rest)=9 ("length (rest)")) -> (substring=w1068:string)
              n1340 = Fract/Exp String To Number(string=w1068) -> (number=w1066:dbl)  [unwired: 3 in, 1 out]
              n1341 = String Subset(string=w1058, offset (0)=25, length (rest)=9 ("length (rest)")) -> (substring=w1064:string)
              n1342 = Fract/Exp String To Number(string=w1064) -> (number=w1062:dbl)  [unwired: 3 in, 1 out]
              n1343 = String Subset(string=w1058, offset (0)=85, length (rest)=9 ("length (rest)")) -> (substring=w1060:string)
              n1344 = Fract/Exp String To Number(string=w1060) -> (number=w1057:dbl)  [unwired: 3 in, 1 out]
            }
            n1345 = for {
              N: w1039 -> [_]
              tunnel: w1054 -> [w1202]
              tunnel: w1053 -> [w1201]
              tunnel: [w1191] -> w966 mode=indexing
              tunnel: [w1189] -> w1023 mode=indexing
              tunnel: [w1190] -> w1018 mode=indexing
              tunnel: w1035 -> [_]
              tunnel: [w1183] -> w1020 mode=indexing
              tunnel: [w1179] -> w989 mode=indexing
              tunnel: [w1175] -> w964 mode=indexing
              tunnel: [w1171] -> w945 mode=indexing
              tunnel: [w1166] -> w905 mode=indexing
              (unwired) TRUE ("line mode (F)")
              # "freq"
              # "Stroke"
              # "Time"
              # "CoF"
              # "Humidity"
              # "Temp"
              # "Air Temp"
              # "ECR"
              n1346 = Read from Text File "Read File"(file (use dialog)=w1202, error in=w1201) -> (text=w1167:string)  [unwired: 2 in, 3 out]
              n1347 = String Subset(string=w1167, offset (0)=0, length (rest)=14 ("length (rest)")) -> (substring=w1195:string)
              n1348 = Fract/Exp String To Number(string=w1195) -> (number=w1191:dbl)  [unwired: 3 in, 1 out]
              n1349 = local write "String 6"(w1167) -> ()
              n1350 = String Subset(string=w1167, offset (0)=15, length (rest)=9 ("length (rest)")) -> (substring=w1198:string)
              n1351 = Fract/Exp String To Number(string=w1198) -> (number=w1189:dbl)  [unwired: 3 in, 1 out]
              n1352 = String Subset(string=w1167, offset (0)=65, length (rest)=9 ("length (rest)")) -> (substring=w1188:string)
              n1353 = Fract/Exp String To Number(string=w1188) -> (number=w1185:dbl)  [unwired: 3 in, 1 out]
              n1354 = Add(x=w1185, y=0.0) -> (x+y=w1183:dbl)
              n1355 = String Subset(string=w1167, offset (0)=35, length (rest)=9 ("length (rest)")) -> (substring=w1192:string)
              n1356 = Fract/Exp String To Number(string=w1192) -> (number=w1190:dbl)  [unwired: 3 in, 1 out]
              n1357 = String Subset(string=w1167, offset (0)=45, length (rest)=9 ("length (rest)")) -> (substring=w1182:string)
              n1358 = Fract/Exp String To Number(string=w1182) -> (number=w1179:dbl)  [unwired: 3 in, 1 out]
              n1359 = String Subset(string=w1167, offset (0)=55, length (rest)=9 ("length (rest)")) -> (substring=w1176:string)
              n1360 = Fract/Exp String To Number(string=w1176) -> (number=w1175:dbl)  [unwired: 3 in, 1 out]
              n1361 = String Subset(string=w1167, offset (0)=25, length (rest)=9 ("length (rest)")) -> (substring=w1174:string)
              n1362 = Fract/Exp String To Number(string=w1174) -> (number=w1171:dbl)  [unwired: 3 in, 1 out]
              n1363 = String Subset(string=w1167, offset (0)=85, length (rest)=9 ("length (rest)")) -> (substring=w1168:string)
              n1364 = Fract/Exp String To Number(string=w1168) -> (number=w1166:dbl)  [unwired: 3 in, 1 out]
            }
            n1365 = Delete From Array(array=w1006, index=0) -> (array with subset deleted=w889:dbl[])  [unwired: 1 in, 1 out]
            n1366 = Delete From Array(array=w998, index=0) -> (array with subset deleted=w887:dbl[])  [unwired: 1 in, 1 out]
            n1367 = Delete From Array(array=w1016, index=0) -> (array with subset deleted=w891:dbl[])  [unwired: 1 in, 1 out]
            n1368 = Delete From Array(array=w996, index=0) -> (array with subset deleted=w976:dbl[])  [unwired: 1 in, 1 out]
            n1369 = Delete From Array(array=w966, index=0) -> (array with subset deleted=w893:dbl[])  [unwired: 1 in, 1 out]
            n1370 = Delete From Array(array=w1004, index=0) -> (array with subset deleted=w977:dbl[])  [unwired: 1 in, 1 out]
            n1371 = Delete From Array(array=w1014, index=0) -> (array with subset deleted=w975:dbl[])  [unwired: 1 in, 1 out]
            n1372 = Delete From Array(array=w1023, index=0) -> (array with subset deleted=w978:dbl[])  [unwired: 1 in, 1 out]
            n1373 = Bundle "Bundle"(w887, w976) -> (w1041:cluster{dbl[], dbl[]})  [unwired: 1 in]
            n1374 = Bundle "Bundle"(w891, w975) -> (w1043:cluster{dbl[], dbl[]})  [unwired: 1 in]
            n1375 = Bundle "Bundle"(w889, w977) -> (w1042:cluster{dbl[], dbl[]})  [unwired: 1 in]
            n1376 = Bundle "Bundle"(w893, w978) -> (w912:cluster{dbl[], dbl[]})  [unwired: 1 in]
            n1377 = Build Array "Build Array"(w912, w1043, w1042, w1041) -> (→"Coefficient Of Friction":cluster{dbl[], dbl[]}[])
            n1378 = Delete From Array(array=w1011, index=0) -> (array with subset deleted=w1012:dbl[])  [unwired: 1 in, 1 out]
            n1379 = Delete From Array(array=w993, index=0) -> (array with subset deleted=w994:dbl[])  [unwired: 1 in, 1 out]
            n1380 = Delete From Array(array=w1002, index=0) -> (array with subset deleted=w1003:dbl[])  [unwired: 1 in, 1 out]
            n1381 = Delete From Array(array=w1020, index=0) -> (array with subset deleted=w1021:dbl[])  [unwired: 1 in, 1 out]
            n1382 = Delete From Array(array=w991, index=0) -> (array with subset deleted=w921:dbl[])  [unwired: 1 in, 1 out]
            n1383 = Delete From Array(array=w1000, index=0) -> (array with subset deleted=w922:dbl[])  [unwired: 1 in, 1 out]
            n1384 = Delete From Array(array=w1018, index=0) -> (array with subset deleted=w924:dbl[])  [unwired: 1 in, 1 out]
            n1385 = Delete From Array(array=w1009, index=0) -> (array with subset deleted=w923:dbl[])  [unwired: 1 in, 1 out]
            n1386 = Bundle "Bundle"(w887, w921) -> (w1033:cluster{dbl[], dbl[]})  [unwired: 1 in]
            n1387 = Bundle "Bundle"(w891, w923) -> (w1034:cluster{dbl[], dbl[]})  [unwired: 1 in]
            n1388 = Bundle "Bundle"(w889, w922) -> (w1032:cluster{dbl[], dbl[]})  [unwired: 1 in]
            n1389 = Bundle "Bundle"(w893, w924) -> (w911:cluster{dbl[], dbl[]})  [unwired: 1 in]
            n1390 = Delete From Array(array=w984, index=0) -> (array with subset deleted=w972:dbl[])  [unwired: 1 in, 1 out]
            n1391 = Build Array "Build Array"(w911, w1034, w1032, w1033) -> (→"Air Temperature":cluster{dbl[], dbl[]}[])
            n1392 = Delete From Array(array=w989, index=0) -> (array with subset deleted=w974:dbl[])  [unwired: 1 in, 1 out]
            "array w/ subset deleted" <- w974
            n1393 = Delete From Array(array=w987, index=0) -> (array with subset deleted=w973:dbl[])  [unwired: 1 in, 1 out]
            n1394 = Delete From Array(array=w964, index=0) -> (array with subset deleted=w920:dbl[])  [unwired: 1 in, 1 out]
            n1395 = Bundle "Bundle"(w887, w994) -> (w1026:cluster{dbl[], dbl[]})  [unwired: 1 in]
            n1396 = Bundle "Bundle"(w891, w1012) -> (w1025:cluster{dbl[], dbl[]})  [unwired: 1 in]
            n1397 = Bundle "Bundle"(w889, w1003) -> (w1027:cluster{dbl[], dbl[]})  [unwired: 1 in]
            n1398 = Bundle "Bundle"(w893, w1021) -> (w885:cluster{dbl[], dbl[]})  [unwired: 1 in]
            n1399 = Build Array "Build Array"(w885, w1025, w1027, w1026) -> (→"XY Graph 13":cluster{dbl[], dbl[]}[])
            n1400 = Delete From Array(array=w983, index=0) -> (array with subset deleted=w971:dbl[])  [unwired: 1 in, 1 out]
            n1401 = Delete From Array(array=w958, index=0) -> (array with subset deleted=w917:dbl[])  [unwired: 1 in, 1 out]
            n1402 = Delete From Array(array=w962, index=0) -> (array with subset deleted=w919:dbl[])  [unwired: 1 in, 1 out]
            n1403 = Delete From Array(array=w960, index=0) -> (array with subset deleted=w918:dbl[])  [unwired: 1 in, 1 out]
            n1404 = call-poly <vilib>:"Mean.vi"("X"=w976) -> ("mean"=→"КОФ4":dbl)  [unwired: 1 out]
            n1405 = call-poly <vilib>:"Mean.vi"("X"=w978) -> ("mean"=→"КОФ1":dbl)  [unwired: 1 out]
            n1406 = call-poly <vilib>:"Mean.vi"("X"=w977) -> ("mean"=→"КОФ3":dbl)  [unwired: 1 out]
            n1407 = Bundle "Bundle"(w893, w974) -> (w907:cluster{dbl[], dbl[]})  [unwired: 1 in]
            n1408 = Bundle "Bundle"(w887, w971) -> (w979:cluster{dbl[], dbl[]})  [unwired: 1 in]
            n1409 = Bundle "Bundle"(w891, w973) -> (w981:cluster{dbl[], dbl[]})  [unwired: 1 in]
            n1410 = Bundle "Bundle"(w889, w972) -> (w980:cluster{dbl[], dbl[]})  [unwired: 1 in]
            n1411 = call-poly <vilib>:"Mean.vi"("X"=w975) -> ("mean"=→"КОФ2":dbl)  [unwired: 1 out]
            n1412 = Build Array "Build Array"(w907, w981, w980, w979) -> (→"Sample Temperature":cluster{dbl[], dbl[]}[])
            n1413 = Bundle "Bundle"(w893, w920) -> (w884:cluster{dbl[], dbl[]})  [unwired: 1 in]
            n1414 = Bundle "Bundle"(w887, w917) -> (w955:cluster{dbl[], dbl[]})  [unwired: 1 in]
            n1415 = Bundle "Bundle"(w891, w919) -> (w957:cluster{dbl[], dbl[]})  [unwired: 1 in]
            n1416 = Bundle "Bundle"(w889, w918) -> (w956:cluster{dbl[], dbl[]})  [unwired: 1 in]
            n1417 = Delete From Array(array=w943, index=0) -> (array with subset deleted=w915:dbl[])  [unwired: 1 in, 1 out]
            n1418 = Delete From Array(array=w941, index=0) -> (array with subset deleted=w914:dbl[])  [unwired: 1 in, 1 out]
            n1419 = call-poly <vilib>:"Mean.vi"("X"=w973) -> ("mean"=→"CP2":dbl)  [unwired: 1 out]
            n1420 = call-poly <vilib>:"Mean.vi"("X"=w971) -> ("mean"=→"CP4":dbl)  [unwired: 1 out]
            n1421 = Build Array "Build Array"(w884, w957, w956, w955) -> (→"Humidity":cluster{dbl[], dbl[]}[])
            n1422 = call-poly <vilib>:"Mean.vi"("X"=w972) -> ("mean"=→"CP3":dbl)  [unwired: 1 out]
            n1423 = call-poly <vilib>:"Mean.vi"("X"=w974) -> ("mean"=→"CP1":dbl)  [unwired: 1 out]
            n1424 = Delete From Array(array=w945, index=0) -> (array with subset deleted=w916:dbl[])  [unwired: 1 in, 1 out]
            n1425 = Bundle "Bundle"(w924, w920) -> (w926:cluster{dbl[], dbl[]})  [unwired: 1 in]
            n1426 = Bundle "Bundle"(w921, w917) -> (w929:cluster{dbl[], dbl[]})  [unwired: 1 in]
            n1427 = Bundle "Bundle"(w923, w919) -> (w927:cluster{dbl[], dbl[]})  [unwired: 1 in]
            n1428 = Bundle "Bundle"(w922, w918) -> (w928:cluster{dbl[], dbl[]})  [unwired: 1 in]
            n1429 = Delete From Array(array=w939, index=0) -> (array with subset deleted=w913:dbl[])  [unwired: 1 in, 1 out]
            n1430 = Build Array "Build Array"(w926, w927, w928, w929) -> (→"Air Temp vs Rh":cluster{dbl[], dbl[]}[])
            n1431 = Build Array "Build Array"(w884, w907) -> (w910:cluster{dbl[], dbl[]}[])
            "XY Graph 17" <- w910
            n1432 = local write "XY Graph 16"(w910) -> ()
            n1433 = Bundle "Bundle"(w891, w915) -> (w937:cluster{dbl[], dbl[]})  [unwired: 1 in]
            n1434 = Bundle "Bundle"(w889, w914) -> (w936:cluster{dbl[], dbl[]})  [unwired: 1 in]
            n1435 = Bundle "Bundle"(w887, w913) -> (w935:cluster{dbl[], dbl[]})  [unwired: 1 in]
            n1436 = Bundle "Bundle"(w893, w916) -> (w938:cluster{dbl[], dbl[]})  [unwired: 1 in]
            n1437 = Delete From Array(array=w905, index=0) -> (array with subset deleted=w892:dbl[])  [unwired: 1 in, 1 out]
            n1438 = Delete From Array(array=w901, index=0) -> (array with subset deleted=w890:dbl[])  [unwired: 1 in, 1 out]
            n1439 = Build Array "Build Array"(w938, w937, w936, w935) -> (→"Stroke":cluster{dbl[], dbl[]}[])
            n1440 = Delete From Array(array=w899, index=0) -> (array with subset deleted=w886:dbl[])  [unwired: 1 in, 1 out]
            n1441 = Delete From Array(array=w900, index=0) -> (array with subset deleted=w888:dbl[])  [unwired: 1 in, 1 out]
            n1442 = Bundle "Bundle"(w893, w892) -> (w898:cluster{dbl[], dbl[]})  [unwired: 1 in]
            n1443 = Bundle "Bundle"(w891, w890) -> (w897:cluster{dbl[], dbl[]})  [unwired: 1 in]
            n1444 = call-poly <vilib>:"Mean.vi"("X"=w916) -> ("mean"=→"КОФ2 2":dbl)  [unwired: 1 out]
            n1445 = Bundle "Bundle"(w887, w886) -> (w895:cluster{dbl[], dbl[]})  [unwired: 1 in]
            n1446 = Bundle "Bundle"(w889, w888) -> (w896:cluster{dbl[], dbl[]})  [unwired: 1 in]
            n1447 = call-poly <vilib>:"Mean.vi"("X"=w915) -> ("mean"=→"КОФ2 3":dbl)  [unwired: 1 out]
            n1448 = call-poly <vilib>:"Mean.vi"("X"=w913) -> ("mean"=→"КОФ2 5":dbl)  [unwired: 1 out]
            n1449 = call-poly <vilib>:"Mean.vi"("X"=w914) -> ("mean"=→"КОФ2 4":dbl)  [unwired: 1 out]
            n1450 = Build Array "Build Array"(w898, w897, w896, w895) -> (→"Frequency":cluster{dbl[], dbl[]}[])
          }
          frame #2 {
          }
          frame #3 {
            n1451 = local read "String Control 4"() -> (w1209:string)
            n1452 = local read "String Control 6"() -> (w1208:string)
            n1453 = local read "String Control 8"() -> (w1207:string)
            n1454 = local read "String Control 2"() -> (w1210:string)
            n1455 = property on="OPEN" class="Bool (strict)"("Visible"=TRUE) -> ()  [unwired: 2 in, 2 out]
            n1456 = Match Pattern(string=w1208, regular expression="Frequency :- ") -> (after substring=w1233:string)  [unwired: 1 in, 3 out]
            n1457 = Match Pattern(string=w1210, regular expression="Frequency :- ") -> (after substring=w1243:string)  [unwired: 1 in, 3 out]
            n1458 = Match Pattern(string=w1209, regular expression="Frequency :- ") -> (after substring=w1238:string)  [unwired: 1 in, 3 out]
            n1459 = Match Pattern(string=w1207, regular expression="Frequency :- ") -> (after substring=w1228:string)  [unwired: 1 in, 3 out]
            n1460 = String Subset(string=w1233, length (rest)=9 ("length (rest)")) -> (substring=w1235:string)  [unwired: 1 in]
            n1461 = String Subset(string=w1243, length (rest)=9 ("length (rest)")) -> (substring=w1245:string)  [unwired: 1 in]
            n1462 = String Subset(string=w1238, length (rest)=9 ("length (rest)")) -> (substring=w1240:string)  [unwired: 1 in]
            n1463 = String Subset(string=w1228, length (rest)=9 ("length (rest)")) -> (substring=w1230:string)  [unwired: 1 in]
            n1464 = Fract/Exp String To Number(string=w1235) -> (number=w1236:dbl)  [unwired: 3 in, 1 out]
            n1465 = Fract/Exp String To Number(string=w1245) -> (number=w1246:dbl)  [unwired: 3 in, 1 out]
            n1466 = Fract/Exp String To Number(string=w1240) -> (number=w1241:dbl)  [unwired: 3 in, 1 out]
            n1467 = Fract/Exp String To Number(string=w1230) -> (number=w1231:dbl)  [unwired: 3 in, 1 out]
            n1468 = local write "freq3"(w1236) -> ()
            n1469 = local write "freq2"(w1241) -> ()
            n1470 = local write "freq1"(w1246) -> ()
            n1471 = local write "freq 4"(w1231) -> ()
            n1472 = local write "Numeric 13"(0 ("Numeric 13")) -> ()
            n1473 = local write "Numeric 11"(0 ("Numeric 11")) -> ()
            n1474 = local write "Numeric 8"(0 ("Numeric 8")) -> ()
            n1475 = local write "Numeric 12"(0 ("Numeric 12")) -> ()
            n1476 = Match Pattern(string=w1208, regular expression="Samples / cycle :- ") -> (after substring=w1216:string)  [unwired: 1 in, 3 out]
            n1477 = Match Pattern(string=w1210, regular expression="Samples / cycle :- ") -> (after substring=w1224:string)  [unwired: 1 in, 3 out]
            n1478 = Match Pattern(string=w1209, regular expression="Samples / cycle :- ") -> (after substring=w1220:string)  [unwired: 1 in, 3 out]
            n1479 = Match Pattern(string=w1207, regular expression="Samples / cycle :- ") -> (after substring=w1212:string)  [unwired: 1 in, 3 out]
            n1480 = String Subset(string=w1216, length (rest)=6 ("length (rest)")) -> (substring=w1218:string)  [unwired: 1 in]
            n1481 = String Subset(string=w1224, length (rest)=6 ("length (rest)")) -> (substring=w1226:string)  [unwired: 1 in]
            n1482 = String Subset(string=w1220, length (rest)=6 ("length (rest)")) -> (substring=w1222:string)  [unwired: 1 in]
            n1483 = String Subset(string=w1212, length (rest)=6 ("length (rest)")) -> (substring=w1214:string)  [unwired: 1 in]
            n1484 = Fract/Exp String To Number(string=w1218) -> (number=w1204:dbl)  [unwired: 3 in, 1 out]
            n1485 = Fract/Exp String To Number(string=w1226) -> (number=w1206:dbl)  [unwired: 3 in, 1 out]
            n1486 = Fract/Exp String To Number(string=w1222) -> (number=w1205:dbl)  [unwired: 3 in, 1 out]
            n1487 = Fract/Exp String To Number(string=w1214) -> (number=w1203:dbl)  [unwired: 3 in, 1 out]
            n1488 = local write "sample2"(w1205) -> ()
            n1489 = local write "sample3"(w1204) -> ()
            n1490 = local write "sample1"(w1206) -> ()
            n1491 = local write "sample4"(w1203) -> ()
          }
        }
      }
    }
    n1492 = Wait (ms)(milliseconds to wait=u32 50) -> ()  [unwired: 1 out]
    n1493 = property on="STOP 3" class="Bool (strict)"() -> ("Visible"=w800:bool)  [unwired: 2 in, 2 out]
    n1494 = case shown="True" w800 {
      frame False {
      }
      frame True {
        n1495 = case shown="True" "Save Results" {
          frame False {
          }
          frame True {
            w1732 = "\r"
            n1496 = local read "Temperature before test"() -> (w1770:dbl)
            n1497 = local read "Temperature after test"() -> (w1772:dbl)
            n1498 = local read "Humidity before test"() -> (w1769:dbl)
            n1499 = local read "Humidity after test"() -> (w1771:dbl)
            n1500 = local read "MWSD"() -> (w1773:dbl)
            n1501 = local read "WS1.4"() -> (w1776:dbl)
            n1502 = local read "AVP"() -> (w1774:dbl)
            n1503 = local read "HCF"() -> (w1775:dbl)
            n1504 = local write "Save Results"(FALSE ("OK Button 5")) -> ()
            n1505 = Number To Fractional String(number=w1772, width (-)=i16 6, precision (6)=i16 1) -> (F-format string=w1750:string)  [unwired: 1 in]
            n1506 = Number To Fractional String(number=w1773, width (-)=i16 6, precision (6)=i16 1) -> (F-format string=w1747:string)  [unwired: 1 in]
            n1507 = Number To Fractional String(number=w1774, width (-)=i16 6, precision (6)=i16 3) -> (F-format string=w1743:string)  [unwired: 1 in]
            n1508 = Number To Fractional String(number=w1771, width (-)=i16 6, precision (6)=i16 1) -> (F-format string=w1754:string)  [unwired: 1 in]
            n1509 = Number To Fractional String(number=w1775, width (-)=i16 6, precision (6)=i16 2) -> (F-format string=w1741:string)  [unwired: 1 in]
            n1510 = Number To Fractional String(number=w1776, width (-)=i16 6, precision (6)=i16 1) -> (F-format string=w1736:string)  [unwired: 1 in]
            n1511 = Number To Fractional String(number=w1770, width (-)=i16 6, precision (6)=i16 1) -> (F-format string=w1758:string)  [unwired: 1 in]
            n1512 = Number To Fractional String(number=w1769, width (-)=i16 6, precision (6)=i16 1) -> (F-format string=w1761:string)  [unwired: 1 in]
            n1513 = local read "String"() -> (w1765:string)
            n1514 = local read "FILE"() -> (w1768:string)
            n1515 = Concatenate Strings(w1765, w1768) -> (w1787:string)
            n1516 = Concatenate Strings(w1787, ".dwm" ("Substring")) -> (w1785:string)
            n1517 = Concatenate Strings(w1741, ")" ("string")) -> (w1739:string)
            n1518 = Concatenate Strings("(" ("string"), w1736, ")Microns" ("string")) -> (w1735:string)
            n1519 = Concatenate Strings("(" ("string"), w1761, " ) % RH," ("string")) -> (w1762:string)
            n1520 = Concatenate Strings("(" ("string"), w1743, ")  kPa," ("string")) -> (w1733:string)
            n1521 = String To Path(string=w1785) -> (path=w1784:path)
